vi "tesla2kA - Hybrid.vi"(1 "SC Current [kA]":dbl format="%.5f", 2 "Magnet Field [T]":dbl=1.0 format="%.4f") -> (0 "Current [kA]":dbl=1.0 format="%.4f")   [LabVIEW 2020]
uses:
  PS Comm Globals.vi
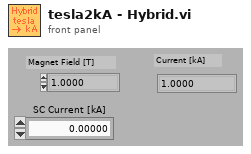
[diagram p1: front panel]
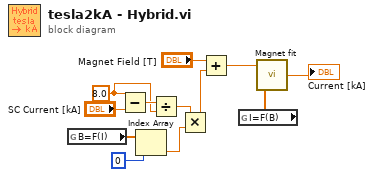
[diagram p0: block diagram]
diagram:
  w4 = 8.0 ("x")
  n1 = global read "PS Comm Globals.vi" "B=F(I)"() -> (w8:dbl[])
  n2 = Subtract(x=w4, y="SC Current [kA]") -> (x-y=w5:dbl)
  n3 = Index Array(array=w8, index=0) -> (element=w2:dbl)
  n4 = Divide(x=w5, y=w4) -> (x/y=w3:dbl)
  n5 = Multiply(x=w3, y=w2) -> (x*y=w1:dbl)
  n6 = Add(x="Magnet Field [T]", y=w1) -> (x+y=w10:dbl)
  n7 = global read "PS Comm Globals.vi" "I=F(B)"() -> (w12:dbl[])
  n8 = call "Magnet fit.vi"("Coefficients"=w12, "Magnet Parameter"=w10) -> ("Conjugate Parameter"=→"Current [kA]":dbl)
